vi "Superior VI Structure Example.vi"   [LabVIEW 2009]
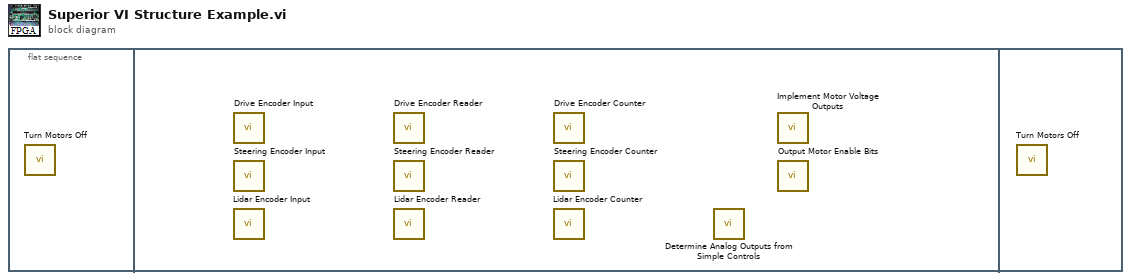
[diagram p0: block diagram]
diagram:
  n1 = flat-sequence {
    frame #0 {
      n2 = call "Turn Motors Off.vi"() -> ()  [unwired: 1 in]
    }
    frame #1 {
      n3 = call "Drive Encoder Input.vi"() -> ()  [unwired: 1 in]
      n4 = call "Steering Encoder Input.vi"() -> ()  [unwired: 1 in]
      n5 = call "Lidar Encoder Input.vi"() -> ()  [unwired: 1 in]
      n6 = call "Drive Encoder Reader.vi"() -> ()  [unwired: 1 in]
      n7 = call "Steering Encoder Reader.vi"() -> ()  [unwired: 1 in]
      n8 = call "Lidar Encoder Reader.vi"() -> ()  [unwired: 1 in]
      n9 = call "Drive Encoder Counter.vi"() -> ()  [unwired: 1 in]
      n10 = call "Steering Encoder Counter.vi"() -> ()  [unwired: 1 in]
      n11 = call "Lidar Encoder Counter.vi"() -> ()  [unwired: 1 in]
      n12 = call "Determine Analog Outputs from Simple Controls.vi"() -> ()  [unwired: 1 in]
      n13 = call "Implement Motor Voltage Outputs.vi"() -> ()  [unwired: 1 in]
      n14 = call "Output Motor Enable Bits.vi"() -> ()  [unwired: 1 in]
    }
    frame #2 {
      n15 = call "Turn Motors Off.vi"() -> ()  [unwired: 1 in]
    }
  }
